vi "VgSweep_Tdep.vi"(8 "Start sweeping":bool) -> ()   [LabVIEW 2015]
uses:
  <vilib>/Utility/file.llb/Read From Spreadsheet File (DBL).vi
panel:
  in  "Record sweep back?":bool
  in  "Stabilisation (min)":i16=10 max=4 step=1
  in  "After measurements:":bool=TRUE
  out "Automatic Mode":i8(ring) items=["OFF", "ON"]
  out "Set Point (T)":dbl
  out "Heater Voltage (V)":dbl
  out "Temperature (K)":dbl
  in  "Custom Folder":string
  out "Communication":string
  in  "Step (T)":dbl=12.0 min=-4.0 max=4.0 step=0.1 format="%.3f"
  out "Experiment ends at:":string
  out "B Array":dbl[](array[numeric])
  in  "Faster":dbl=10.0
  in  "HigherRate?":bool
  out "Hours":dbl format="%.1f"
  out "Estimated time of experiment:":i16
  out "# of connections":i16=1 min=-4 max=4 step=1
  in  "Final T (K)":dbl=12.0 min=-4.0 max=4.0 step=0.1 format="%.3f"
  in  "Initial T (K)":dbl min=-4.0 max=4.0 step=0.1 format="%.3f"
  in  "V2:":dbl=1.0 min=-4.0 max=4.0 step=0.1 format="%.3f"
  in  "Sweep rate , V/min":dbl=0.6 min=0.0 max=1.0 step=0.01 format="%.4f"
  in  "V1:":dbl min=-4.0 max=4.0 step=0.1 format="%.3f"
  # "Define interval of gate voltage\nfor main Keithley 2400 (address 12):"
  # "Set temperatures at which sweeps\nare made"
  # "Go to Initial T?"
  # "min."
  # "="
  # "hours"
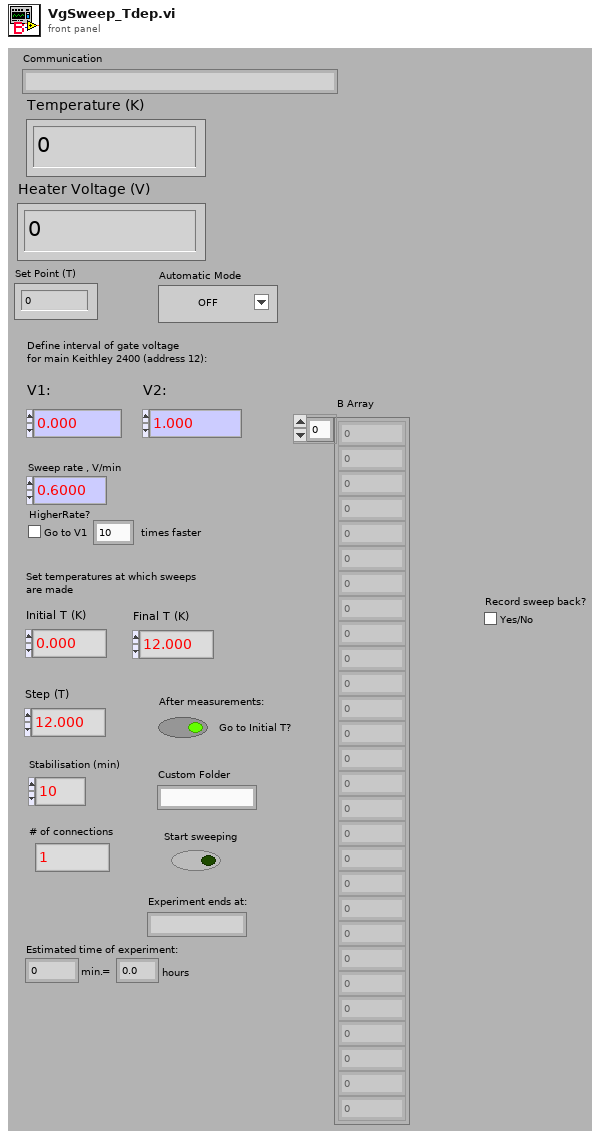
[diagram p1: front panel]
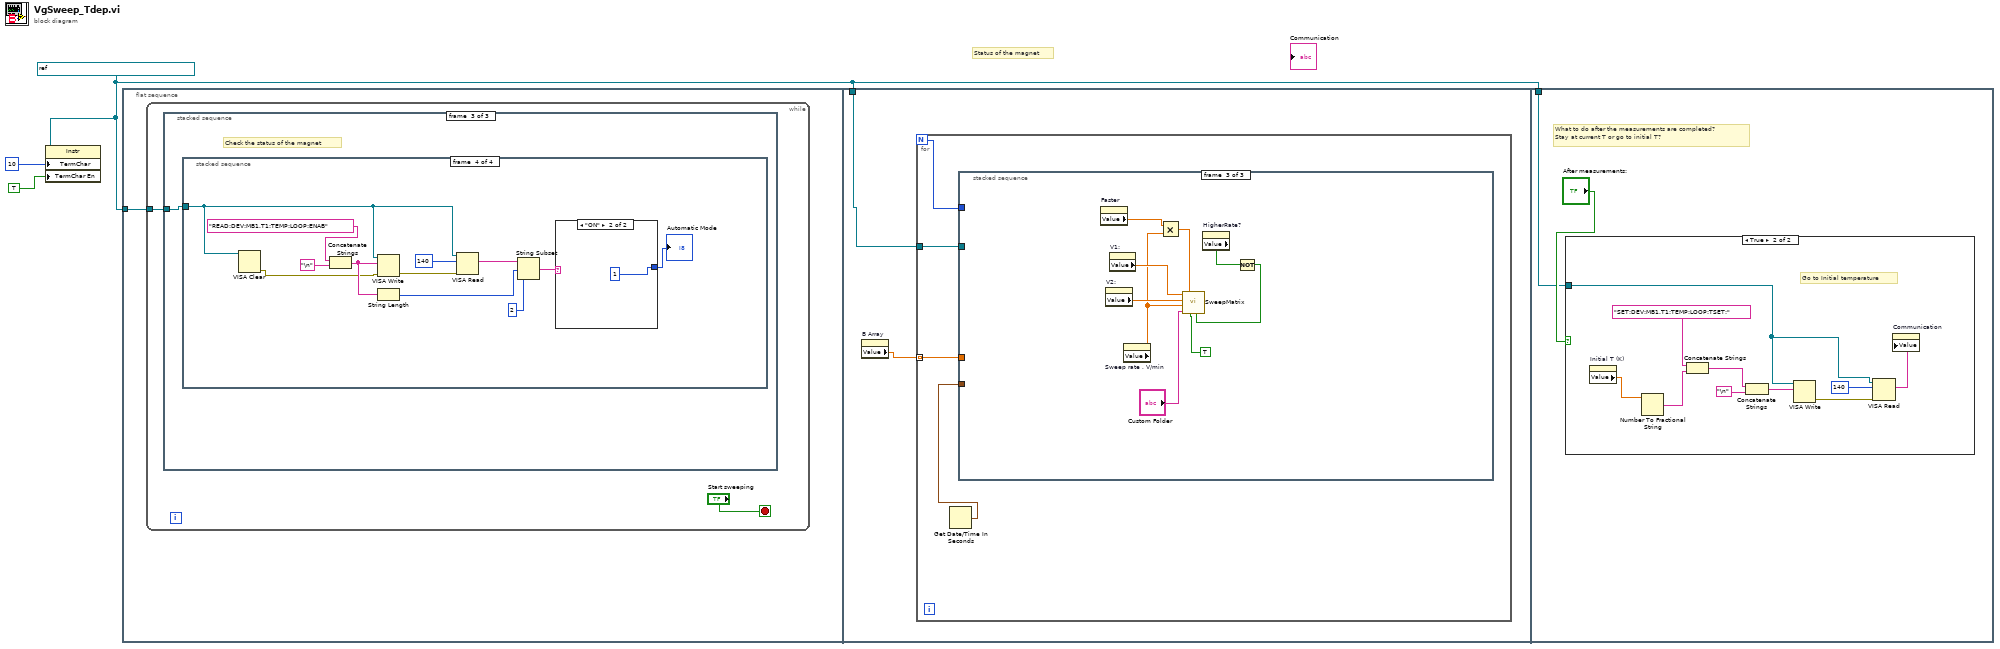
[diagram p0: block diagram]
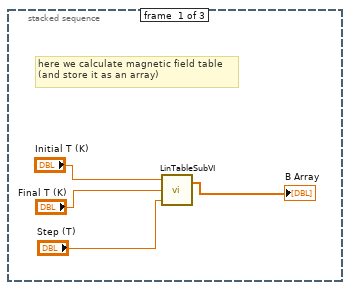
[diagram p2: hidden frame]
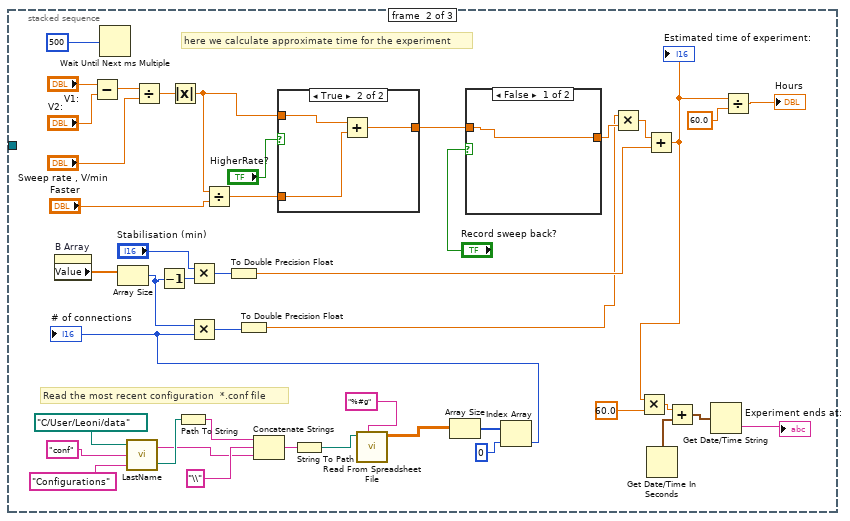
[diagram p3: hidden frame]
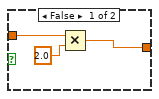
[diagram p4: hidden frame]
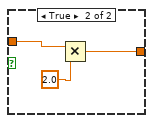
[diagram p5: hidden frame]
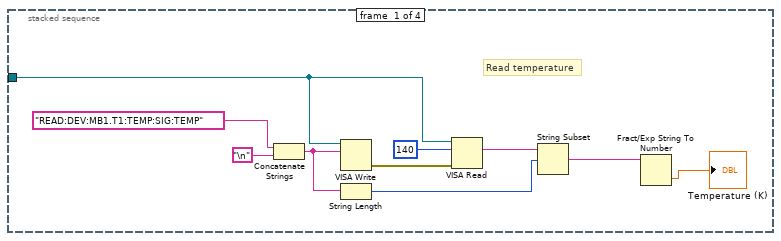
[diagram p6: hidden frame]
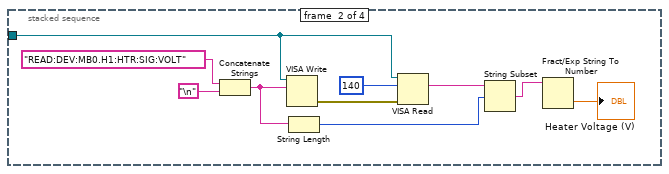
[diagram p7: hidden frame]
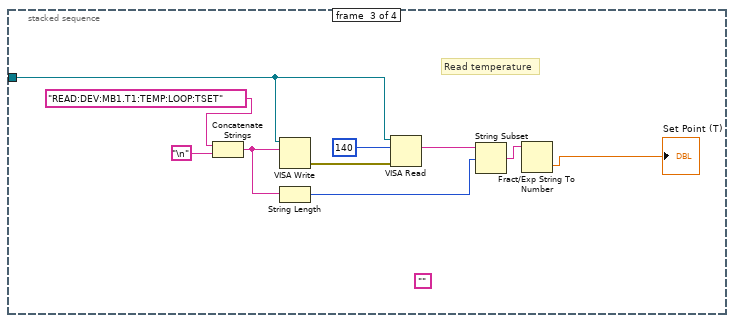
[diagram p8: hidden frame]
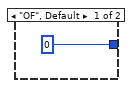
[diagram p9: hidden frame]
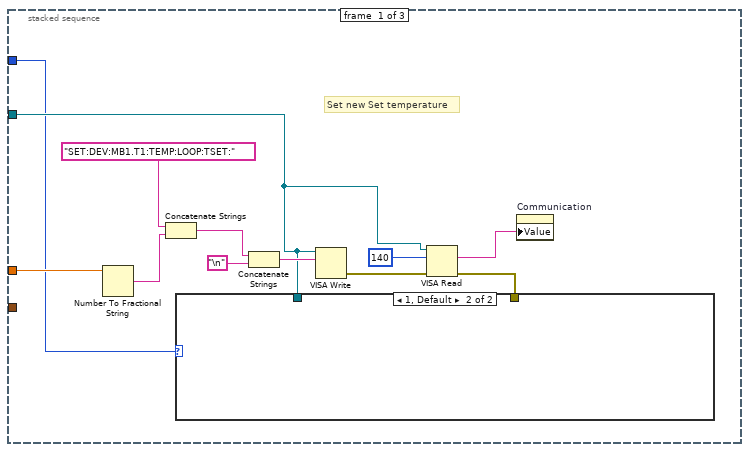
[diagram p10: hidden frame]
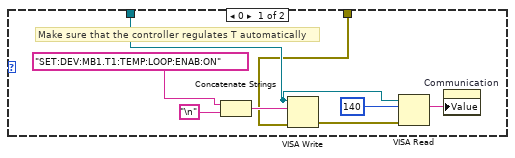
[diagram p11: hidden frame]
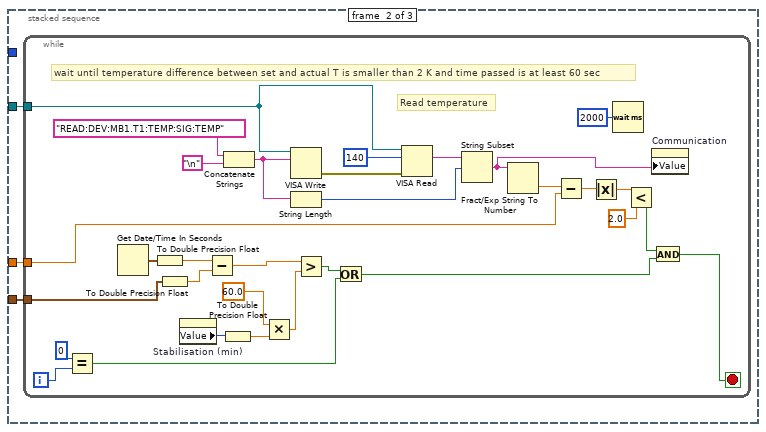
[diagram p12: hidden frame]
diagram:
  w1 = refnum<visa-resource-name> "TCPIP0::192.168.128.2::7020::SOCKET" ("VISA resource name")
  # "Status of the magnet"
  n1 = property class="Instr"(reference=w1, "TermChar"=10, "TermChar En"=TRUE) -> ()  [unwired: 1 in, 2 out]
  n2 = flat-sequence {
    tunnel: w1 -> [w4]
    tunnel: w1 -> [w111]
    tunnel: w1 -> [w179]
    frame #0 {
      n3 = while {
        tunnel: w4 -> [w5]
        stop <- "Start sweeping" stop-if-true
        n4 = stacked-sequence {
          tunnel: w5 -> [_ _ w65]
          frame #0 {
            # "here we calculate magnetic field table\n(and store it as an array)"
            n5 = call "LinTableSubVI.vi"("Step"="Step (T)", "Final"="Final T (K)", "Initial"="Initial T (K)") -> ("Array"=→"B Array":dbl[])  [unwired: 1 in]
          }
          frame #1 {
            # "Read the most recent configuration  *.conf file"
            # "here we calculate approximate time for the experiment"
            n6 = property on="B Array" class="Arr (strict)"() -> ("Value"=w41:dbl[])  [unwired: 2 in, 2 out]
            n7 = Subtract(x="V1:", y="V2:") -> (x-y=w54:dbl)
            n8 = Wait Until Next ms Multiple(millisecond multiple=500) -> ()  [unwired: 1 out]
            n9 = Array Size(array=w41) -> (size(s)=w25:i32)
            n10 = call "LastName.vi"("Custom Folder"="Configurations", "Extention"="conf", "User Data Folder"=path "C:/User/Leoni/data") -> ("created path"=w36:path, "String"=w35:string)
            n11 = Divide(x=w54, y="Sweep rate , V/min") -> (x/y=w53:dbl)
            n12 = Decrement(x=w25) -> (x-1=w26:i32)
            n13 = Absolute Value(x=w53) -> (abs(x)=w16:dbl)
            n14 = Path To String(path=w36) -> (string=w40:string)
            n15 = Multiply(x="Stabilisation (min)", y=w26) -> (x*y=w22:i32)
            n16 = Divide(x=w16, y="Faster") -> (x/y=w17:dbl)
            n17 = To Double Precision Float(number=w22) -> (double precision float=w21:dbl)
            n18 = Concatenate Strings(w40, "\\", w35) -> (w38:string)
            n19 = case shown="True" "HigherRate?" {
              tunnel: [w55 w60] -> w18
              tunnel: w17 -> [_ w59]
              tunnel: w16 -> [w56 w58]
              frame False {
                n20 = Multiply(x=w56, y=2.0) -> (x*y=w55:dbl)
              }
              frame True {
                n21 = Add(x=w58, y=w59) -> (x+y=w60:dbl)
              }
            }
            n22 = String To Path(string=w38) -> (path=w31:path)
            n23 = call-poly <vilib>:"Read From Spreadsheet File.vi"("format (%.3f)"="%#g", "file path (dialog if empty)"=w31) -> ("all rows"=w28:dbl[][])  [unwired: 5 in, 4 out]
            n24 = Array Size(array=w28) -> (size(s)=w30:i32[])
            n25 = case shown="False" "Record sweep back?" {
              tunnel: w18 -> [w61 w63]
              tunnel: [w61 w62] -> w14
              frame False {
              }
              frame True {
                n26 = Multiply(x=w63, y=2.0) -> (x*y=w62:dbl)
              }
            }
            n27 = Index Array(array=w30, index=0) -> (element=w27:i32)
            "# of connections" <- w27
            n28 = Multiply(x=w25, y=w27) -> (x*y=w12:i32)
            n29 = To Double Precision Float(number=w12) -> (double precision float=w11:dbl)
            n30 = Multiply(x=w11, y=w14) -> (x*y=w13:dbl)
            n31 = Add(x=w13, y=w21) -> (x+y=w23:dbl)
            "Estimated time of experiment:" <- w23
            n32 = Multiply(x=w23, y=60.0) -> (x*y=w45:dbl)
            n33 = Get Date/Time In Seconds() -> (seconds since 1Jan1904=w44:timestamp)
            n34 = Add(x=w45, y=w44) -> (x+y=w43:timestamp)
            n35 = Get Date/Time String(seconds (now)=w43) -> (time string=→"Experiment ends at:":string)  [unwired: 2 in, 1 out]
            n36 = Divide(x=w23, y=60.0) -> (x/y=→"Hours":dbl)
          }
          frame #2 {
            # "Check the status of the magnet"
            n37 = stacked-sequence {
              tunnel: w65 -> [w66 w76 w86 w97]
              frame #0 {
                # "Read temperature"
                n38 = Concatenate Strings("READ:DEV:MB1.T1:TEMP:SIG:TEMP" ("string"), "\n") -> (w68:string)
                n39 = VISA Write(VISA resource name=w66, write buffer=w68) -> (error out=w74:errorcluster)  [unwired: 1 in, 2 out]
                n40 = String Length(string=w68) -> (length=w69:i32)
                n41 = VISA Read(VISA resource name=w66, byte count=140, error in (no error)=w74) -> (read buffer=w70:string)  [unwired: 3 out]
                n42 = String Subset(string=w70, offset (0)=w69) -> (substring=w67:string)  [unwired: 1 in]
                n43 = Fract/Exp String To Number(string=w67) -> (number=→"Temperature (K)":dbl)  [unwired: 3 in, 1 out]
              }
              frame #1 {
                n44 = Concatenate Strings("READ:DEV:MB0.H1:HTR:SIG:VOLT" ("string"), "\n") -> (w80:string)
                n45 = VISA Write(VISA resource name=w76, write buffer=w80) -> (error out=w84:errorcluster)  [unwired: 1 in, 2 out]
                n46 = String Length(string=w80) -> (length=w78:i32)
                n47 = VISA Read(VISA resource name=w76, byte count=140, error in (no error)=w84) -> (read buffer=w79:string)  [unwired: 3 out]
                n48 = String Subset(string=w79, offset (0)=w78) -> (substring=w77:string)  [unwired: 1 in]
                n49 = Fract/Exp String To Number(string=w77) -> (number=→"Heater Voltage (V)":dbl)  [unwired: 3 in, 1 out]
              }
              frame #2 {
                (unwired) ""
                # "Read temperature"
                n50 = Concatenate Strings("READ:DEV:MB1.T1:TEMP:LOOP:TSET" ("string"), "\n") -> (w88:string)
                n51 = VISA Write(VISA resource name=w86, write buffer=w88) -> (error out=w94:errorcluster)  [unwired: 1 in, 2 out]
                n52 = String Length(string=w88) -> (length=w89:i32)
                n53 = VISA Read(VISA resource name=w86, byte count=140, error in (no error)=w94) -> (read buffer=w90:string)  [unwired: 3 out]
                n54 = String Subset(string=w90, offset (0)=w89) -> (substring=w87:string)  [unwired: 1 in]
                n55 = Fract/Exp String To Number(string=w87) -> (number=→"Set Point (T)":dbl)  [unwired: 3 in, 1 out]
              }
              frame #3 {
                n56 = VISA Clear(VISA resource name=w97) -> (error out=w96:errorcluster)  [unwired: 1 in, 1 out]
                n57 = Concatenate Strings("READ:DEV:MB1.T1:TEMP:LOOP:ENAB" ("string"), "\n") -> (w101:string)
                n58 = VISA Write(VISA resource name=w97, write buffer=w101, error in (no error)=w96) -> (error out=w107:errorcluster)  [unwired: 2 out]
                n59 = String Length(string=w101) -> (length=w102:i32)
                n60 = VISA Read(VISA resource name=w97, byte count=140, error in (no error)=w107) -> (read buffer=w103:string)  [unwired: 3 out]
                n61 = String Subset(string=w103, offset (0)=w102, length (rest)=2) -> (substring=w100:string)
                n62 = case shown="\"ON\"" w100 {
                  tunnel: [0 1] -> w99
                  frame "OF", Default {
                  }
                  frame "ON" {
                  }
                }
                "Automatic Mode" <- w99
              }
            }
          }
        }
      }
    }
    frame #1 {
      n63 = property on="B Array" class="Arr (strict)"() -> ("Value"=w110:dbl[])  [unwired: 2 in, 2 out]
      n64 = for {
        N -> [w112]
        tunnel: w111 -> [w115]
        tunnel: w110 -> [w114] mode=indexing
        n65 = Get Date/Time In Seconds() -> (seconds since 1Jan1904=w113:timestamp)
        n66 = stacked-sequence {
          tunnel: w115 -> [w118 w138 _]
          tunnel: w114 -> [w120 w137 _]
          tunnel: w113 -> [_ w136 _]
          tunnel: w112 -> [w116 _ _]
          frame #0 {
            # "Set new Set temperature"
            n67 = Number To Fractional String(number=w120) -> (F-format string=w122:string)  [unwired: 3 in]
            n68 = Concatenate Strings("SET:DEV:MB1.T1:TEMP:LOOP:TSET:" ("string"), w122) -> (w127:string)
            n69 = Concatenate Strings(w127, "\n") -> (w126:string)
            n70 = VISA Write(VISA resource name=w118, write buffer=w126) -> (error out=w123:errorcluster)  [unwired: 1 in, 2 out]
            n71 = VISA Read(VISA resource name=w118, byte count=140, error in (no error)=w123) -> (read buffer=w121:string, error out=w117:errorcluster)  [unwired: 2 out]
            n72 = case shown="1, Default" w116 {
              tunnel: w118 -> [w130 _]
              tunnel: w117 -> [w129 _]
              frame 0 {
                # "Make sure that the controller regulates T automatically"
                n73 = Concatenate Strings("SET:DEV:MB1.T1:TEMP:LOOP:ENAB:ON" ("string"), "\n") -> (w132:string)
                n74 = VISA Write(VISA resource name=w130, write buffer=w132, error in (no error)=w129) -> (error out=w135:errorcluster)  [unwired: 2 out]
                n75 = VISA Read(VISA resource name=w130, byte count=140, error in (no error)=w135) -> (read buffer=w128:string)  [unwired: 3 out]
                n76 = property on="Communication" class="Str"("Value"=w128) -> ()  [unwired: 2 in, 2 out]
              }
              frame 1, Default {
              }
            }
            n77 = property on="Communication" class="Str"("Value"=w121) -> ()  [unwired: 2 in, 2 out]
          }
          frame #1 {
            n78 = while {
              tunnel: w138 -> [w162]
              tunnel: w137 -> [w160]
              tunnel: w136 -> [w155]
              i -> [w147]
              stop <- w150 stop-if-true
              # "wait until temperature difference between set and actual T is smaller than 2 K and time passed is at least 60 sec"
              # "Read temperature"
              n79 = Equal?(x=0, y=w147) -> (x = y?=w144:bool)
              n80 = Get Date/Time In Seconds() -> (seconds since 1Jan1904=w156:timestamp)
              n81 = To Double Precision Float(number=w156) -> (double precision float=w154:dbl)
              n82 = To Double Precision Float(number=w155) -> (double precision float=w153:dbl)
              n83 = property on="Stabilisation (min)" class="DigNum (strict)"() -> ("Value"=w142:i16)  [unwired: 2 in, 2 out]
              n84 = Subtract(x=w154, y=w153) -> (x-y=w152:dbl)
              n85 = To Double Precision Float(number=w142) -> (double precision float=w141:dbl)
              n86 = Concatenate Strings("READ:DEV:MB1.T1:TEMP:SIG:TEMP" ("string"), "\n") -> (w163:string)
              n87 = Multiply(x=60.0, y=w141) -> (x*y=w139:dbl)
              n88 = VISA Write(VISA resource name=w162, write buffer=w163) -> (error out=w169:errorcluster)  [unwired: 1 in, 2 out]
              n89 = String Length(string=w163) -> (length=w164:i32)
              n90 = Greater?(x=w152, y=w139) -> (0:w145:bool)
              n91 = Or(x=w145, y=w144) -> (x .or. y?=w143:bool)
              n92 = VISA Read(VISA resource name=w162, byte count=140, error in (no error)=w169) -> (read buffer=w165:string)  [unwired: 3 out]
              n93 = String Subset(string=w165, offset (0)=w164) -> (substring=w148:string)  [unwired: 1 in]
              n94 = Fract/Exp String To Number(string=w148) -> (number=w161:dbl)  [unwired: 3 in, 1 out]
              n95 = Subtract(x=w161, y=w160) -> (x-y=w159:dbl)
              n96 = Absolute Value(x=w159) -> (abs(x)=w158:dbl)
              n97 = Wait (ms)(milliseconds to wait=2000) -> ()  [unwired: 1 out]
              n98 = Less?(x=w158, y=2.0) -> (x < y?=w151:bool)
              n99 = property on="Communication" class="Str"("Value"=w148) -> ()  [unwired: 2 in, 2 out]
              n100 = And(x=w151, y=w143) -> (x .and. y?=w150:bool)
            }
          }
          frame #2 {
            n101 = property on="Faster" class="DigNum (strict)"() -> ("Value"=w173:dbl)  [unwired: 2 in, 2 out]
            n102 = property on="V2:" class="DigNum (strict)"() -> ("Value"=w177:dbl)  [unwired: 2 in, 2 out]
            n103 = property on="V1:" class="DigNum (strict)"() -> ("Value"=w176:dbl)  [unwired: 2 in, 2 out]
            n104 = property on="Sweep rate , V/min" class="DigNum (strict)"() -> ("Value"=w172:dbl)  [unwired: 2 in, 2 out]
            n105 = Multiply(x=w173, y=w172) -> (x*y=w171:dbl)
            n106 = property on="HigherRate?" class="Bool (strict)"() -> ("Value"=w174:bool)  [unwired: 2 in, 2 out]
            n107 = Not(x=w174) -> (.not. x?=w170:bool)
            n108 = call "SweepMatrix.vi"("From V2 to V1"=w170, "Play Button"=TRUE, "Rate w/o measure, V/min"=w171, "Custom Folder"="Custom Folder", "Sweep rate, V/min"=w172, "V2 (V)"=w177, "V1 (V)"=w176) -> ()  [unwired: 5 in]
          }
        }
      }
    }
    frame #2 {
      # "What to do after the measurements are completed?\nStay at current T or go to initial T?"
      n109 = case shown="True" "After measurements:" {
        tunnel: w179 -> [_ w182]
        frame False {
          # "Stay at current T"
        }
        frame True {
          # "Go to Initial temperature"
          n110 = property on="Initial T (K)" class="DigNum (strict)"() -> ("Value"=w183:dbl)  [unwired: 2 in, 2 out]
          n111 = Number To Fractional String(number=w183) -> (F-format string=w185:string)  [unwired: 3 in]
          n112 = Concatenate Strings("SET:DEV:MB1.T1:TEMP:LOOP:TSET:" ("string"), w185) -> (w190:string)
          n113 = Concatenate Strings(w190, "\n") -> (w189:string)
          n114 = VISA Write(VISA resource name=w182, write buffer=w189) -> (error out=w186:errorcluster)  [unwired: 1 in, 2 out]
          n115 = VISA Read(VISA resource name=w182, byte count=140, error in (no error)=w186) -> (read buffer=w181:string)  [unwired: 3 out]
          n116 = property on="Communication" class="Str"("Value"=w181) -> ()  [unwired: 2 in, 2 out]
        }
      }
    }
  }
